vi "Refresh If Required.vi"(8 "error in (no error)":errorcluster, 11 "Ethernet in":refnum<class "ENET_BS120x.lvclass">) -> (0 "error out":errorcluster, 3 "Ethernet out":refnum<class "ENET_BS120x.lvclass">)   [LabVIEW 2021, in "BS120x Driver.lvlib" / "ENET_BS120x.lvclass"]
uses:
  ENET_BS120x.lvclass
  ENET_BS120x.lvclass/ENET_BS120x.ctl
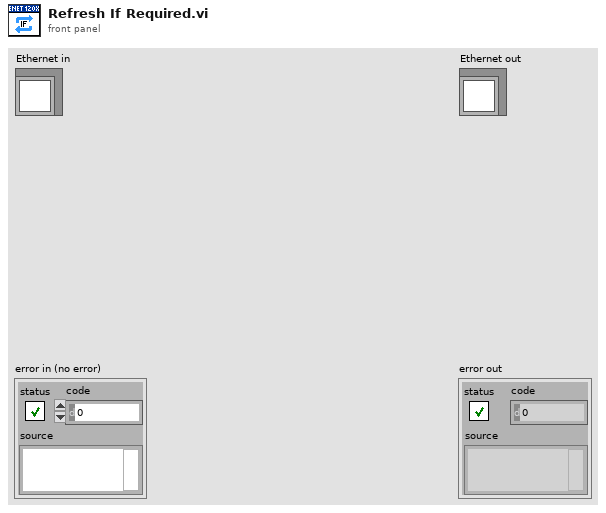
[diagram p1: front panel]
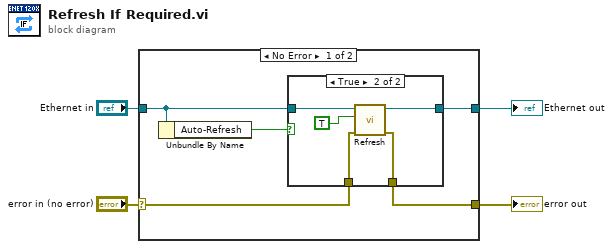
[diagram p0: block diagram]
diagram:
  n1 = case shown="No Error" "error in (no error)" {
    selector: "error in (no error)" -> [w8 w18]
    tunnel: [w7 w18] -> w3
    tunnel: [w9 w17] -> w1
    tunnel: "Ethernet in" -> [w6 w17]
    frame No Error {
      n2 = Unbundle By Name(w6) -> ("Auto-Refresh"=w5:bool)
      n3 = case shown="True" w5 {
        tunnel: [w10 w16] -> w9
        tunnel: w8 -> [w11 w15]
        tunnel: [w11 w14] -> w7
        tunnel: w6 -> [w10 w12]
        frame False {
        }
        frame True {
          n4 = call "Refresh.vi"("error in (no error)"=w15, "Force Refresh (F)"=TRUE, "Ethernet in"=w12) -> ("error out"=w14:errorcluster, "Ethernet out"=w16:refnum<class "ENET_BS120x.lvclass">)  [unwired: 7 in]
        }
      }
    }
    frame Error {
    }
  }
  "error out" <- w3
  "Ethernet out" <- w1
